vi "Czuj_odl_zmiana2.vi"() -> ()   [LabVIEW 2021]
uses:
  VISA.ctl
  stop.ctl
  Meter.ctl
  chart.ctl
  Control 1.ctl
  Unit.ctl
  <vilib>/Instr/_visa.llb/VISA Configure Serial Port (Instr).vi
panel:
  in  "Choose unit:":T1
  out "Distance:":T2
  out "Waveform Chart":T3
  out "Meter":T4 scale=0.0..1000.0
  in  "stop":T5
  in  "VISA resource name":T6
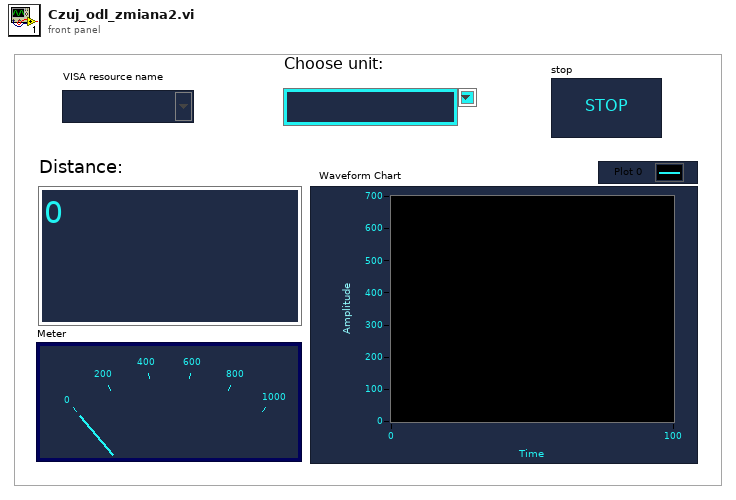
[diagram p1: front panel]
types:
  T1 = typedef "Unit.ctl" = string
  T2 = typedef "Control 1.ctl" = dbl
  T3 = typedef "chart.ctl" = dbl
  T4 = typedef "Meter.ctl" = dbl
  T5 = typedef "stop.ctl" = bool
  T6 = typedef "VISA.ctl" = refnum<visa-resource-name>
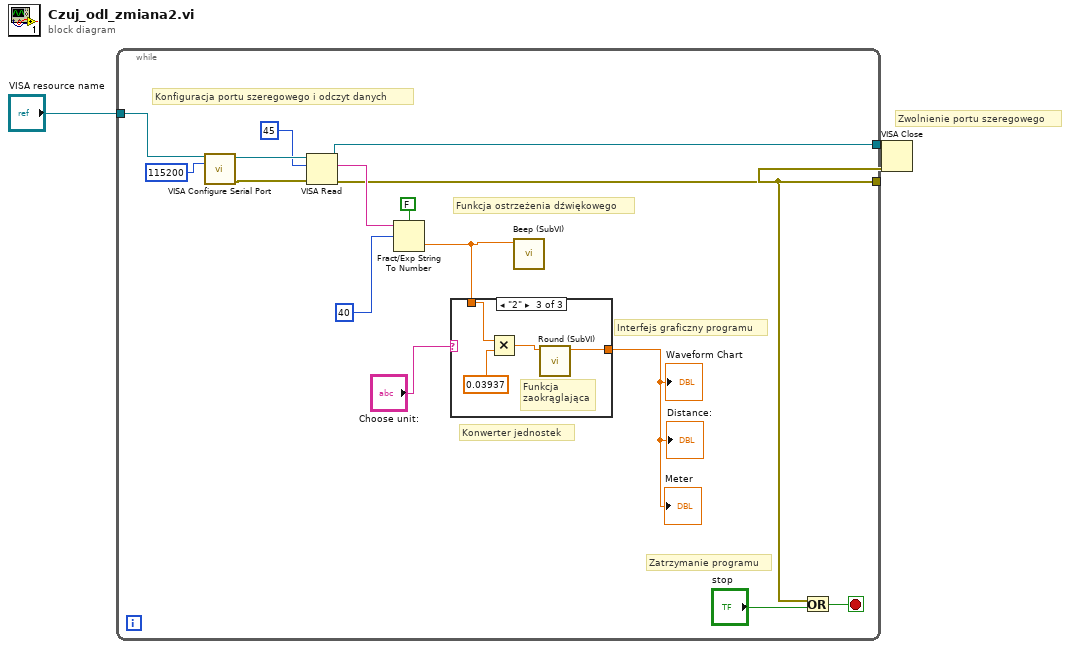
[diagram p0: block diagram]
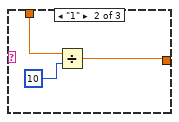
[diagram p3: hidden frame]
diagram:
  # "Zwolnienie portu szeregowego"
  n1 = while {
    tunnel: "VISA resource name" -> [w18]
    tunnel: [w16] -> w2
    tunnel: [w7] -> w1
    stop <- w9 stop-if-true
    # "Zatrzymanie programu"
    # "Konwerter jednostek"
    # "Funkcja ostrzeżenia dźwiękowego"
    # "Interfejs graficzny programu"
    # "Konfiguracja portu szeregowego i odczyt danych"
    n2 = call-poly "VISA Configure Serial Port"("VISA resource name"=w18, "baud rate (9600)"=u32 115200) -> ("VISA resource name out"=w17:refnum<visa-resource-name>, "error out"=w10:errorcluster)  [unwired: 12 in]
    n3 = VISA Read(VISA resource name=w17, byte count=u32 45, error in (no error)=w10) -> (VISA resource name out=w16:refnum<visa-resource-name>, read buffer=w13:string, error out=w7:errorcluster)  [unwired: 1 out]
    n4 = Fract/Exp String To Number(use system decimal point (T)=FALSE, string=w13, offset=40) -> (number=w5:dbl)  [unwired: 1 in, 1 out]
    n5 = case shown="\"2\"" "Choose unit:" {
      tunnel: [w19 w22 w23] -> w6
      tunnel: w5 -> [w19 w21 w26]
      frame "0", Default {
      }
      frame "1" {
        n6 = Divide(x=w21, y=10) -> (x/y=w22:dbl)
      }
      frame "2" {
        # "Funkcja\nzaokrąglająca"
        n7 = Multiply(x=w26, y=0.03937) -> (x*y=w24:dbl)
        n8 = call "Round (SubVI).vi"("Numeric in"=w24) -> ("Numeric out"=w23:dbl)  [unwired: 10 in]
      }
    }
    "Meter" <- w6
    "Waveform Chart" <- w6
    "Distance:" <- w6
    n9 = call "Beep (SubVI).vi"("Numeric"=w5) -> ()  [unwired: 11 in]
    n10 = Or(x=w7, y="stop") -> (x .or. y?=w9:T5)
  }
  n11 = VISA Close(VISA resource name=w2, error in (no error)=w1) -> ()  [unwired: 1 out]
